vi "StopAndWaitForIdle.vi"(7 "forceStop (f)":bool, 11 "error in (no error)":errorcluster) -> (3 "error out":errorcluster)   [LabVIEW 2018, in "AnalysisModule.lvlib"]
uses:
  AnalysisModule.lvlib
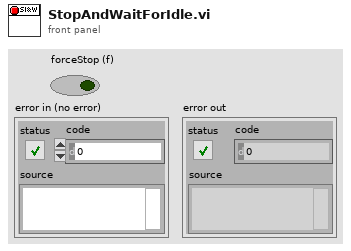
[diagram p1: front panel]
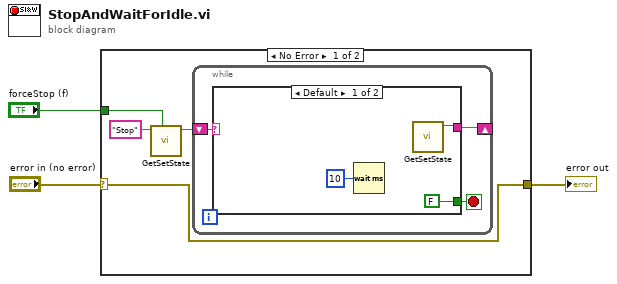
[diagram p0: block diagram]
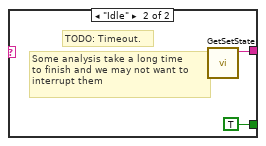
[diagram p2: hidden frame]
diagram:
  n1 = case shown="No Error" "error in (no error)" {
    selector: "error in (no error)" -> [w4 w16]
    tunnel: "forceStop (f)" -> [w7 _]
    tunnel: [w4 w16] -> w1
    frame No Error {
      n2 = call "GetSetState.vi"("Set (f)"=w7, "State In"="Stop") -> ("State Out"=w5:string)  [unwired: 9 in]
      n3 = while {
        shift-right: [w9] -> _
        shift-left: w5 -> [w10]
        stop <- w8 stop-if-true
        n4 = case shown="Default" w10 {
          tunnel: [w11 w15] -> w9
          tunnel: [FALSE TRUE] -> w8
          frame Default {
            n5 = Wait (ms)(milliseconds to wait=u32 10) -> ()  [unwired: 1 out]
            n6 = call "GetSetState.vi"() -> ("State Out"=w11:string)  [unwired: 11 in]
          }
          frame "Idle" {
            # "Some analysis take a long time\nto finish and we may not want to \ninterrupt them"
            # "TODO: Timeout."
            n7 = call "GetSetState.vi"() -> ("State Out"=w15:string)  [unwired: 11 in]
          }
        }
      }
    }
    frame Error {
    }
  }
  "error out" <- w1
